vi "CleanUp.vi"(0 "object in":refnum<class "Cleanup.lvclass">, 5 "error in (no error)":errorcluster) -> (14 "object out":refnum<class "Cleanup.lvclass">, 19 "error out":errorcluster)   [LabVIEW 2022 SP3, in "Cleanup.lvclass"]
uses:
  Cleanup.lvclass
  Role_class/Role.lvclass
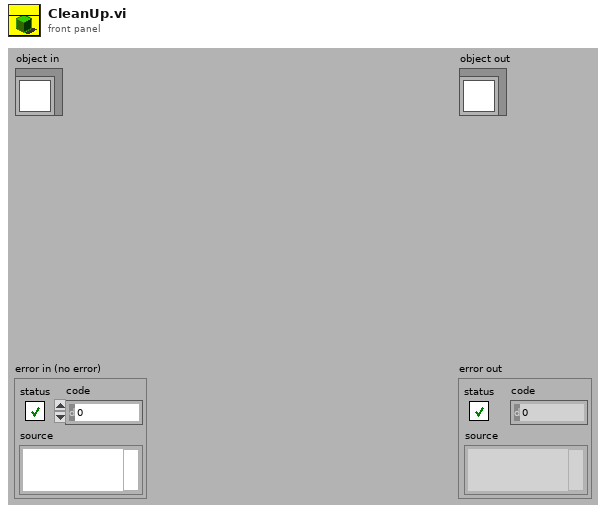
[diagram p1: front panel]
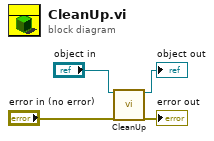
[diagram p0: block diagram]
diagram:
  n1 = call-parent "CleanUp.vi"("object in"="object in", "error in (no error)"="error in (no error)") -> ("object out"=→"object out":refnum<class "Cleanup.lvclass">, "error out"=→"error out":errorcluster)  [unwired: 16 in]
